vi "rsemi_trace_scan_fetch.vi"() -> ()   [LabVIEW 2015]
uses:
  <instrlib>/Rohde&Schwarz EMI Test Receiver/Rohde&Schwarz EMI Test Receiver.lvlib
panel:
  in  "Stop Frequency Range 3":dbl=2000000000.0 caption="Stop Frequency Range 2" format="%#.9p"
  in  "Start Frequency Range 3":dbl=1400000000.0 caption="Start Frequency Range 2" format="%#.9p"
  in  "VISA resource name":refnum<visa-resource-name>="TCPIP::10.102.100.41::INST"
  in  "Reset":bool=TRUE
  in  "Stop Frequency Range 2":dbl=1400000000.0 format="%#.9p"
  in  "Start Frequency Range 2":dbl=500000000.0 format="%#.9p"
  in  "Stop Frequency Range 1":dbl=500000000.0 format="%#.9p"
  in  "Start Frequency Range 1":dbl=100000000.0 format="%#.9p"
  out "Spectrum Graph":cluster{dbl[], dbl[]}(graph)
  # "Example to perform the sweep scan on a R&S EMI Receiver. \nThe scan ranges are set to a fixed number or 3 (2 are default).\nTo run the example, adjust the VISA resource name to fit your instrument."
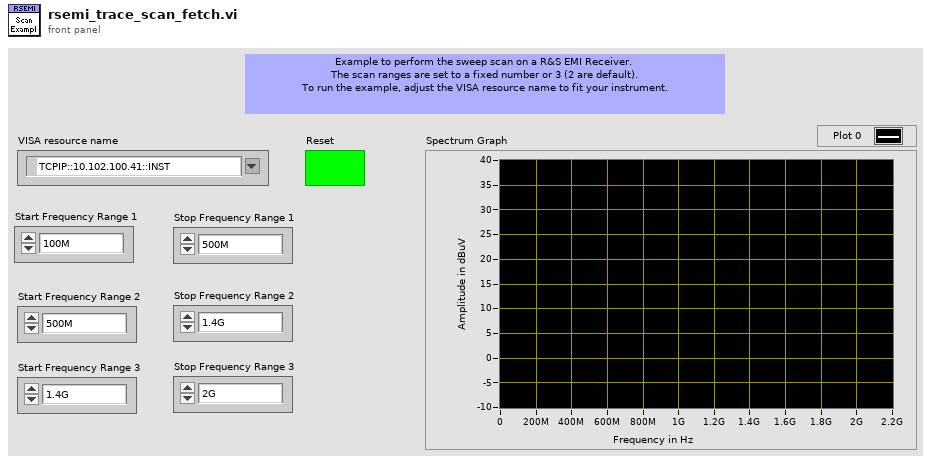
[diagram p1: front panel]
types:
  T1 = cluster{"Start Frequency Range 1":dbl, "Frequency Scan Step Size":dbl, "Stop Frequency Range 1":dbl}
  T2 = cluster{"Start Frequency Range 2":dbl, "Frequency Scan Step Size":dbl, "Stop Frequency Range 2":dbl}
  T3 = cluster{"Start Frequency Range 2":dbl, "Frequency Scan Step Size":dbl, "Stop Frequency Range 2":dbl}[]
  T4 = cluster{"Start Frequency Range 3":dbl, "Frequency Scan Step Size":dbl, "Stop Frequency Range 3":dbl}
  T5 = cluster{"Start Frequency Range 3":dbl, "Frequency Scan Step Size":dbl, "Stop Frequency Range 3":dbl}[]
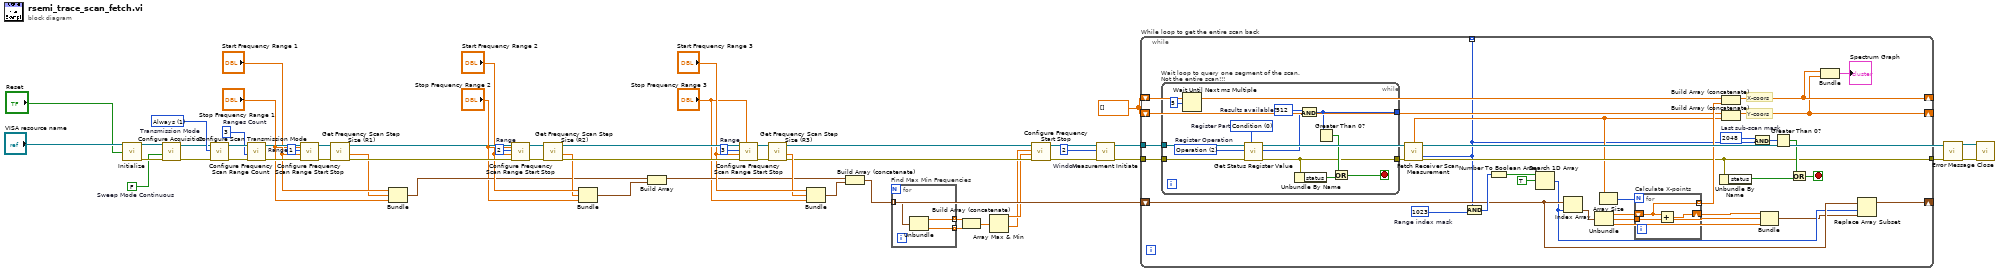
[diagram p0: block diagram]
diagram:
  w24 = 3  # Ranges Count
  w25 = 3  # Range
  w32 = 2  # Range
  w42 = 1  # Range
  w43 = dbl[] []
  w47 = 2  # Window
  w50 = FALSE  # Sweep Mode Continuous
  w56 = 1 items=["Never", "Always", "Clickrate Analyze"]  # Transmission Mode
  n1 = call <instrlib>:"Initialize.vi"("VISA resource name"="VISA resource name", "Reset (T)"="Reset") -> ("VISA resource name out"=w52:refnum<visa-resource-name>, "error out"=w53:errorcluster)  [unwired: 12 in]
  n2 = call <instrlib>:"Configure Acquisition.vi"("error in (no error)"=w53, "Sweep Mode Continuous (F)"=w50, "VISA resource name"=w52) -> ("error out"=w55:errorcluster, "VISA resource name out"=w54:refnum<visa-resource-name>)  [unwired: 7 in]
  n3 = call <instrlib>:"Configure Scan Transmission Mode.vi"("error in (no error)"=w55, "Transmission Mode (Never)"=w56, "VISA resource name"=w54) -> ("error out"=w31:errorcluster, "VISA resource name out"=w30:refnum<visa-resource-name>)  [unwired: 7 in]
  n4 = call <instrlib>:"Configure Frequency Scan Range Count.vi"("error in (no error)"=w31, "Ranges Count (0)"=w24, "VISA resource name"=w30) -> ("error out"=w29:errorcluster, "VISA resource name out"=w28:refnum<visa-resource-name>)  [unwired: 7 in]
  n5 = call <instrlib>:"Configure Frequency Scan Range Start Stop.vi"("Stop Frequency (30.0e6)"="Stop Frequency Range 1", "error in (no error)"=w29, "Start Frequency (150.0e3)"="Start Frequency Range 1", "Range (1)"=w42, "VISA resource name"=w28) -> ("error out"=w40:errorcluster, "VISA resource name out"=w39:refnum<visa-resource-name>)  [unwired: 5 in]
  n6 = call "Get Frequency Scan Step Size (R1)"("error in (no error)"=w40, "instrument handle"=w39) -> ("error out"=w38:errorcluster, "Frequency Scan Step Size"=w22:dbl, "instrument handle out"=w37:refnum<visa-resource-name>)  [unwired: 7 in]
  n7 = Bundle("Start Frequency Range 1"="Start Frequency Range 1", "Frequency Scan Step Size"=w22, "Stop Frequency Range 1"="Stop Frequency Range 1") -> (w17:T1)  [unwired: 1 in]
  n8 = call <instrlib>:"Configure Frequency Scan Range Start Stop.vi"("Stop Frequency (30.0e6)"="Stop Frequency Range 2", "error in (no error)"=w38, "Start Frequency (150.0e3)"="Start Frequency Range 2", "Range (1)"=w32, "VISA resource name"=w37) -> ("error out"=w36:errorcluster, "VISA resource name out"=w35:refnum<visa-resource-name>)  [unwired: 5 in]
  n9 = call "Get Frequency Scan Step Size (R2)"("error in (no error)"=w36, "instrument handle"=w35) -> ("error out"=w27:errorcluster, "Frequency Scan Step Size"=w20:dbl, "instrument handle out"=w26:refnum<visa-resource-name>)  [unwired: 7 in]
  n10 = Bundle("Start Frequency Range 2"="Start Frequency Range 2", "Frequency Scan Step Size"=w20, "Stop Frequency Range 2"="Stop Frequency Range 2") -> (w16:T2)  [unwired: 1 in]
  n11 = Build Array(w17, w16) -> (w15:T3)
  n12 = call <instrlib>:"Configure Frequency Scan Range Start Stop.vi"("Stop Frequency (30.0e6)"="Stop Frequency Range 3", "error in (no error)"=w27, "Start Frequency (150.0e3)"="Start Frequency Range 3", "Range (1)"=w25, "VISA resource name"=w26) -> ("error out"=w34:errorcluster, "VISA resource name out"=w33:refnum<visa-resource-name>)  [unwired: 5 in]
  n13 = call "Get Frequency Scan Step Size (R3)"("error in (no error)"=w34, "instrument handle"=w33) -> ("error out"=w13:errorcluster, "Frequency Scan Step Size"=w18:dbl, "instrument handle out"=w12:refnum<visa-resource-name>)  [unwired: 7 in]
  n14 = Bundle("Start Frequency Range 3"="Start Frequency Range 3", "Frequency Scan Step Size"=w18, "Stop Frequency Range 3"="Stop Frequency Range 3") -> (w14:T4)  [unwired: 1 in]
  n15 = Build Array (concatenate)(w15, w14) -> (w6:T5)
  n16 = for "Find Max Min Frequencies" {
    tunnel: w6 -> [w59] mode=indexing
    tunnel: [w58] -> w5 mode=indexing
    tunnel: [w57] -> w4 mode=indexing
    n17 = Unbundle(w59) -> ("Start Frequency Range 3"=w58:dbl, "Stop Frequency Range 3"=w57:dbl)  [unwired: 1 out]
  }
  n18 = Build Array (concatenate)(w5, w4) -> (w3:dbl[])
  n19 = Array Max & Min(array=w3) -> (max value=w2:dbl, min value=w1:dbl)  [unwired: 2 out]
  n20 = call <instrlib>:"Configure Frequency Start Stop.vi"("error in (no error)"=w13, "Stop Frequency (fmax)"=w2, "Start Frequency (0.0)"=w1, "VISA resource name"=w12) -> ("error out"=w11:errorcluster, "VISA resource name out"=w10:refnum<visa-resource-name>)  [unwired: 6 in]
  n21 = call <instrlib>:"Measurement Initiate.vi"("error in (no error)"=w11, "Window (1)"=w47, "VISA resource name"=w10) -> ("error out"=w45:errorcluster, "VISA resource name out"=w46:refnum<visa-resource-name>)  [unwired: 7 in]
  n22 = while "While loop to get the entire scan back" {
    tunnel: w46 -> [w88]
    tunnel: w45 -> [w90]
    tunnel: [w77] -> w44
    shift-right: [w75] -> _
    shift-left: w43 -> [w82]
    shift-right: [w74] -> _
    shift-left: w43 -> [w80]
    shift-right: [w68] -> _
    shift-left: w6 -> [w67]
    tunnel: [w62] -> _ mode=indexing
    stop <- w84 stop-if-true
    w78 = 1023  # Range index mask
    w86 = 2048  # Last sub-scan mask
    # "Y-coors"
    # "X-coors"
    n23 = while "Wait loop to query one segment of the scan. Not the entire scan!!!" {
      tunnel: w88 -> [w104]
      tunnel: w90 -> [w105]
      tunnel: [w99] -> _
      tunnel: [w95] -> w89
      stop <- w96 stop-if-true
      w101 = 512  # Results available?
      w102 = 0 items=["Condition", "Event"]  # Register Part
      w103 = 2 items=["Questionable"=1, "Operation"=2]  # Register Operation
      n24 = Wait Until Next ms Multiple(millisecond multiple=u32 5) -> ()  [unwired: 1 out]
      n25 = call <instrlib>:"Get Status Register Value.vi"("Register Part (Event)"=w102, "error in (no error)"=w105, "Register Operation (Questionable)"=w103, "VISA resource name"=w104) -> ("error out"=w95:errorcluster, "Register Value"=w100:i32)  [unwired: 5 in, 1 out]
      n26 = Unbundle By Name(w95) -> ("status"=w98:bool)
      n27 = And(x=w101, y=w100) -> (x .and. y?=w99:i32)
      n28 = Greater Than 0?(x=w99) -> (x > 0?=w97:bool)
      n29 = Or(x=w97, y=w98) -> (x .or. y?=w96:bool)
    }
    n30 = call <instrlib>:"Fetch Receiver Scan Measurement.vi"("VISA resource name"=w88, "error in (no error)"=w89) -> ("Result of Trace 1"=w76:dbl[], "Trace Status"=w62:i32, "error out"=w77:errorcluster)  [unwired: 6 in, 5 out]
    n31 = And(x=w62, y=w78) -> (x .and. y?=w73:i32)
    n32 = Number To Boolean Array(number=w73) -> (Boolean array=w72:bool[])
    n33 = Search 1D Array(1D array=w72, element=TRUE) -> (index of element=w66:i32)  [unwired: 1 in]
    n34 = Index Array(array=w67, index=w66) -> (element=w70:T4)
    n35 = Unbundle(w70) -> ("Start Frequency Range 3"=w69:dbl, "Frequency Scan Step Size"=w64:dbl, "Stop Frequency Range 3"=w60:dbl)
    n36 = Array Size(array=w76) -> (size(s)=w61:i32)
    n37 = for "Calculate X-points" {
      N: w61 -> [_]
      tunnel: [w91] -> w81 mode=indexing
      shift-right: [w92] -> w63
      shift-left: w69 -> [w91]
      tunnel: w64 -> [w93]
      n38 = Add(x=w91, y=w93) -> (x+y=w92:dbl)
    }
    n39 = Unbundle By Name(w77) -> ("status"=w87:bool)
    n40 = Build Array (concatenate)(w82, w81) -> (w75:dbl[])
    n41 = Build Array (concatenate)(w80, w76) -> (w74:dbl[])
    n42 = And(x=w86, y=w62) -> (x .and. y?=w85:i32)
    n43 = Bundle("Start Frequency Range 3"=w63, "Frequency Scan Step Size"=w64, "Stop Frequency Range 3"=w60) -> (w65:T4)  [unwired: 1 in]
    n44 = Greater Than 0?(x=w85) -> (x > 0?=w83:bool)
    n45 = Or(x=w83, y=w87) -> (x .or. y?=w84:bool)
    n46 = Bundle(w75, w74) -> (→"Spectrum Graph":cluster{dbl[], dbl[]})  [unwired: 1 in]
    n47 = Replace Array Subset(array=w67, new element=w65, index=w66) -> (w68:T5)
  }
  n48 = call <instrlib>:"Error Message.vi"("VISA resource name"=w46, "error in (no error)"=w44) -> ("VISA resource name out"=w48:refnum<visa-resource-name>, "error out"=w49:errorcluster)  [unwired: 9 in, 3 out]
  n49 = call <instrlib>:"Close.vi"("error in (no error)"=w49, "VISA resource name"=w48) -> ()  [unwired: 9 in, 1 out]
